vi "Main.vi"() -> ()   [LabVIEW 2019]
uses:
  <vilib>/sound2/lvsound2.llb/Sound Data Format.ctl
panel:
  out "error out":errorcluster
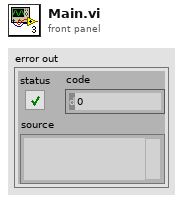
[diagram p1: front panel]
types:
  T1 = typedef "Sound Data Format.ctl" = cluster{"sample rate (S/s)":dbl, "number of channels":i32, "bits per sample":i32}
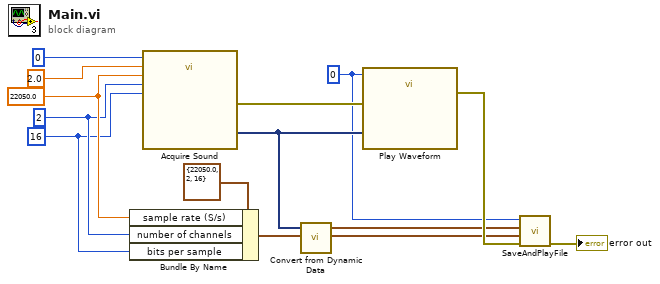
[diagram p0: block diagram]
diagram:
  w1 = u32 0 ("Device")
  w6 = 16 ("Resolution (bits)")
  w7 = 2 ("#Channels")
  w8 = 22050.0 ("Sample rate (Hz)")
  n1 = Bundle By Name(cluster=T1 {"sample rate (S/s)"=22050.0, "number of channels"=2, "bits per sample"=16} ("Sound Format"), "sample rate (S/s)"=w8, "number of channels"=w7, "bits per sample"=w6) -> (w5:T1)
  n2 = call "Acquire Sound"("Device"=u32 0, "Duration (s)"=2.0, "Sample rate (Hz)"=w8, "#Channels"=w7, "Resolution (bits)"=w6) -> ("Data"=w3:dynamicdata, "error out"=w13:errorcluster)  [unwired: 13 in]
  n3 = call "Convert from Dynamic Data"("Dynamic Data Type"=w3) -> ("Array of Waveform"=w2:waveform(dbl)[])  [unwired: 3 in]
  n4 = call "Play Waveform"("Device"=w1, "Data"=w3, "error in"=w13) -> ("error out"=w10:errorcluster)  [unwired: 16 in]
  n5 = call "SaveAndPlayFile.vi"("error in (no error)"=w10, "Sound Format"=w5, "Waveform(s) in"=w2, "Speaker device ID"=w1) -> ("error out"=→"error out":errorcluster)  [unwired: 7 in]
